vi "Create Stream.vi"(8 "error in (no error)":errorcluster, 10 "TCP Connection":refnum<k5>, 11 "TCP Client in":refnum<class "TCP Client.lvclass">) -> (0 "error out":errorcluster, 3 "TCP Client out":refnum<class "TCP Client.lvclass">)   [LabVIEW 2020, in "Stream-TCP.lvlib" / "TCP Client.lvclass"]
uses:
  TCP Client.lvclass
  TCP Client.lvclass/TCP Client.ctl
  TCP Stream/TCP Stream.lvclass
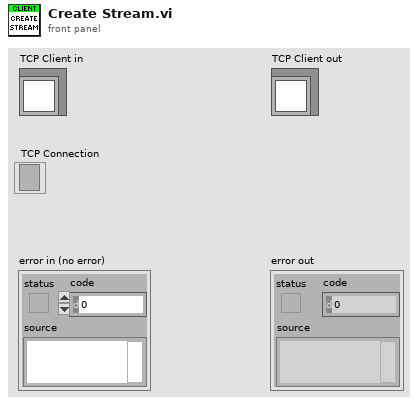
[diagram p1: front panel]
types:
  T1 = typedef "Stream-TCP.lvlib/Client Command Queue.ctl" = refnum<queue>
  T2 = typedef "Stream-TCP.lvlib/TCP Mode.ctl" = enum16{"buffered", "raw"}
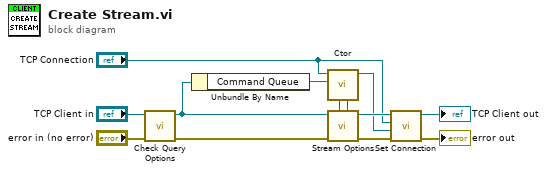
[diagram p0: block diagram]
diagram:
  n1 = call "Check Query Options.vi"("error in (no error)"="error in (no error)", "TCP Client in"="TCP Client in") -> ("error out"=w8:errorcluster, "TCP Client out"=w7:refnum<class "TCP Client.lvclass">)  [unwired: 8 in]
  n2 = Unbundle By Name(w7) -> ("Command Queue"=w12:T1)
  n3 = call "Stream Options.vi"("error in (no error)"=w8, "TCP Client in"=w7) -> ("error out"=w4:errorcluster, "TCP Client out"=w13:refnum<class "TCP Client.lvclass">, "Timeout ms"=w6:i32, "TCP Mode"=w5:T2)  [unwired: 6 in]
  n4 = call "Ctor.vi"("Timeout ms"=w6, "TCP Mode"=w5, "Client Command Queue"=w12, "TCP Connection"="TCP Connection") -> ("TCP Stream out"=w11:refnum<class "TCP Stream.lvclass">)  [unwired: 6 in, 1 out]
  n5 = call "Set Connection.vi"("error in (no error)"=w4, "TCP Stream"=w11, "TCP Connection"="TCP Connection", "TCP Client in"=w13) -> ("error out"=→"error out":errorcluster, "TCP Client out"=→"TCP Client out":refnum<class "TCP Client.lvclass">)  [unwired: 6 in]
